vi "irP.vi"(8 "error in (no error)":errorcluster, 11 "目標":dbl) -> (0 "error out":errorcluster, 3 "公分":dbl(slide) scale=0.0..200.0)   [LabVIEW 2019]
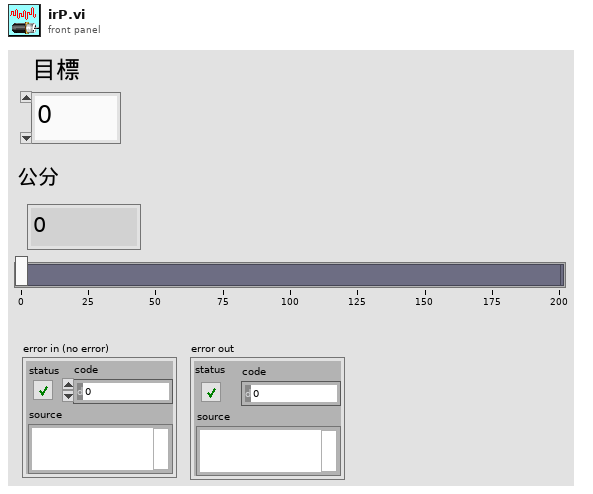
[diagram p1: front panel]
types:
  T1 = enum16{"請選擇紅外線", "紅外線1", "紅外線2", "紅外線3", "紅外線4", "紅外線5", "紅外線6", "紅外線7", "紅外線8"}
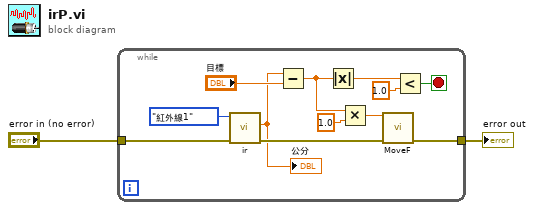
[diagram p0: block diagram]
diagram:
  n1 = while {
    tunnel: "error in (no error)" -> [w5]
    tunnel: [w7] -> w1
    stop <- w8 stop-if-true
    n2 = call "ir.vi"("error in (no error)"=w5, "選擇紅外線"=T1."紅外線1") -> ("error out"=w4:errorcluster, "公分"=w3:dbl)  [unwired: 8 in]
    "公分" <- w3
    n3 = Subtract(x=w3, y="目標") -> (x-y=w11:dbl)
    n4 = Absolute Value(x=w11) -> (abs(x)=w10:dbl)
    n5 = Multiply(x=w11, y=1.0) -> (x*y=w12:dbl)
    n6 = call "MoveF.vi"("X"=w12, "error in (no error)"=w4) -> ("error out"=w7:errorcluster)  [unwired: 13 in]
    n7 = Less?(x=w10, y=1.0) -> (x < y?=w8:bool)
  }
  "error out" <- w1
